vi "Axial Scanning Selector.vi"(11 "Axial Scan":enum16{"OFF", "ON"}(ring)) -> (2 "D(linear - [], nonlinear [0,0]":dbl[](array[numeric]))   [LabVIEW 2017]
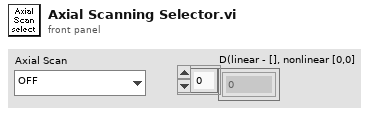
[diagram p1: front panel]
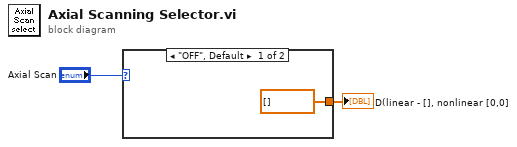
[diagram p0: block diagram]
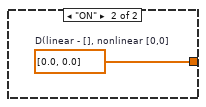
[diagram p2: hidden frame]
diagram:
  n1 = case shown="\"OFF\", Default" "Axial Scan" {
    tunnel: [dbl[] [] ("D(linear - [], nonlinear [0,0]") w4] -> w1
    frame "OFF", Default {
    }
    frame "ON" {
      w4 = dbl[] [0.0, 0.0]  # D(linear - [], nonlinear [0,0]
    }
  }
  "D(linear - [], nonlinear [0,0]" <- w1
